vi "CLASS - Generate2DTrain.vi"(8 "error in":errorcluster, 11 "Local":T6={"Parameters"={"Plot"=refnum, "Data"={"Split"={"X Train"=[], "X Test"=[], "Y Train"=[], "Y Test"=[]}, "Predict"=[]}, "Display"={"Choice"=enum."All", "Indexe"={"X"=0, "Y"=0}}, "Property"={"Train Style"=enum."Full circle", "Test OK Style"=enum."Full square", "Label Color"=[8978528, 4367871, 1985280], "Test NO OK"={"Style"=enum."Cross", "Color"=16716800}}}, "2D Array"=[], "Rating 2D Array"=[], "Point ID"=[], "GoodPredict"=0}) -> (0 "error out":errorcluster, 3 "Local Out":T6)   [LabVIEW 2020]
doc: "Generate 2D graph"
uses:
  Controls/2DParameters.ctl
  _Controls/Datas.ctl
  _Controls/PointPropertyMultipleLabel.ctl
  _Controls/Style.ctl
  _Controls/2DData.ctl
types:
  T1 = typedef "2DParameters.ctl" = cluster{"Plot":refnum<vi>, "Data":T2, "Display":cluster{"Choice":enum16{"All", "Train", "Test"}, "Indexe":cluster{"X":i32, "Y":i32}}, "Property":T3}
  T2 = typedef "Datas.ctl" = cluster{"Split":cluster{"X Train":dbl[][], "X Test":dbl[][], "Y Train":dbl[][], "Y Test":dbl[][]}, "Predict":dbl[][]}
  T3 = typedef "PointPropertyMultipleLabel.ctl" = cluster{"Train Style":T4, "Test OK Style":T4, "Label Color":u32[], "Test NO OK":cluster{"Style":T4, "Color":u32}}
  T4 = typedef "Style.ctl" = enum16{"Empty circle", "Full circle", "Empty square", "Full square", "Cross"}
  T5 = typedef "2DData.ctl" = cluster{"Tag":i32, "X":dbl[], "Y":dbl[]}
  T6 = cluster{"Parameters":T1, "2D Array":cluster{"X":dbl[], "Y":dbl[]}[], "Rating 2D Array":T5[], "Point ID":cluster{"DataUse":enum16{"Dataset", "Train", "Test"}, "Color":u32}[], "GoodPredict":i32}
  T7 = cluster{"DataUse":enum16{"Dataset", "Train", "Test"}, "Color":u32}
  T8 = cluster{"X Train":dbl[][], "X Test":dbl[][], "Y Train":dbl[][], "Y Test":dbl[][]}
  T9 = cluster{"DataUse":enum16{"Dataset", "Train", "Test"}, "Color":u32}[]
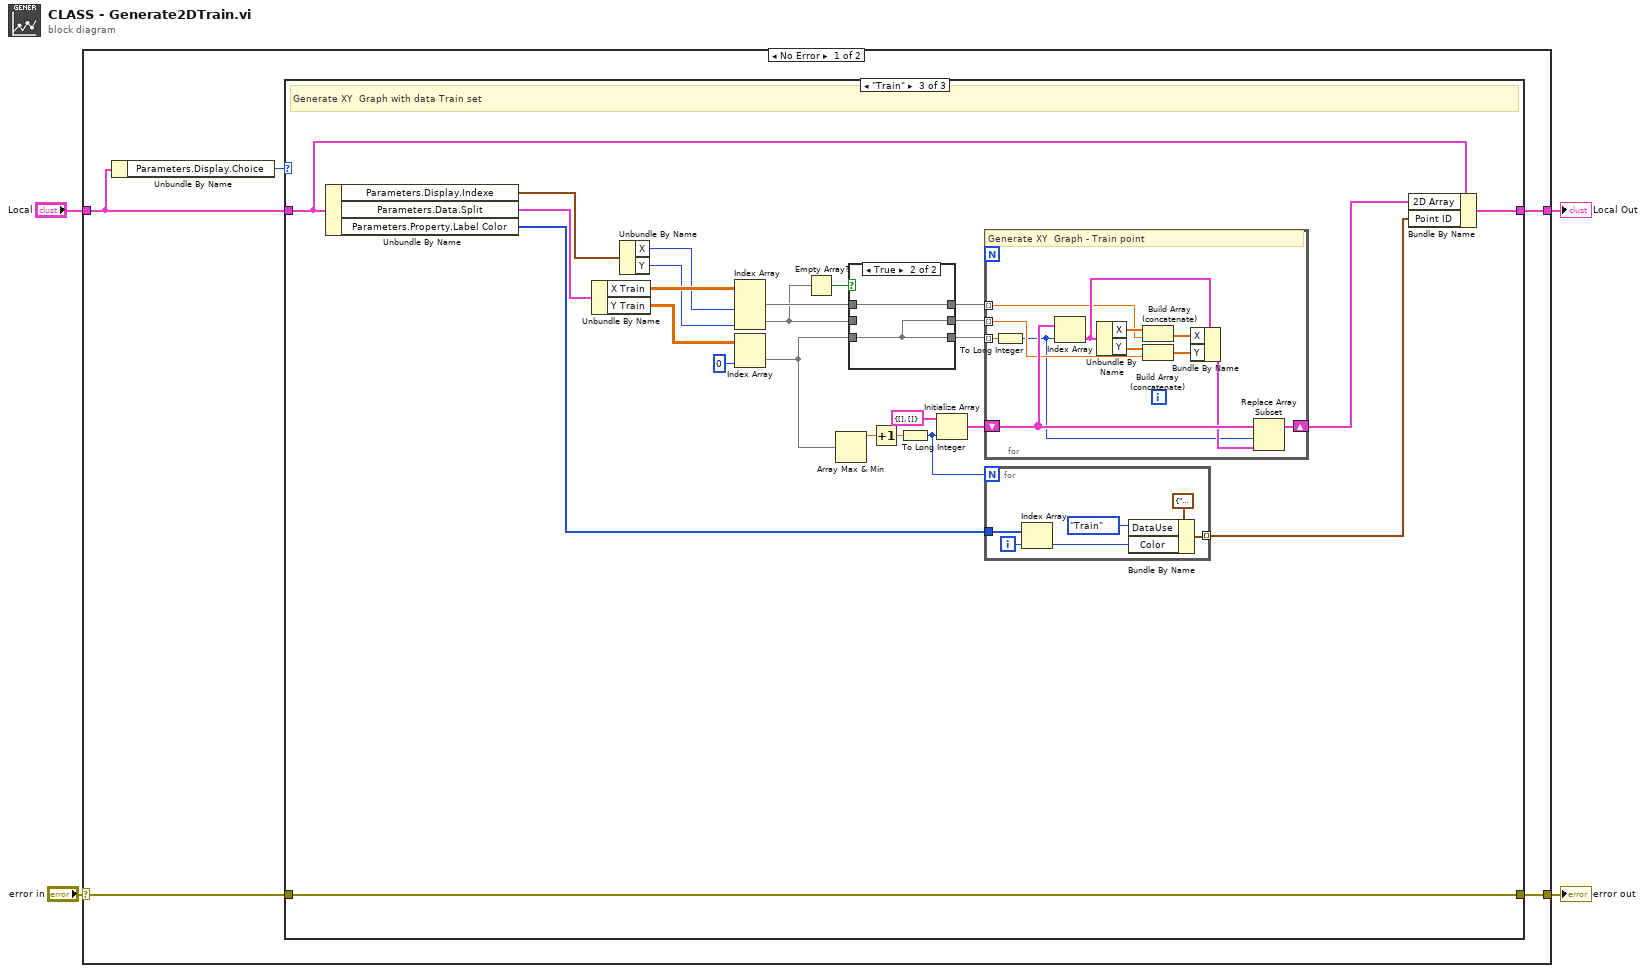
[diagram p0: block diagram]
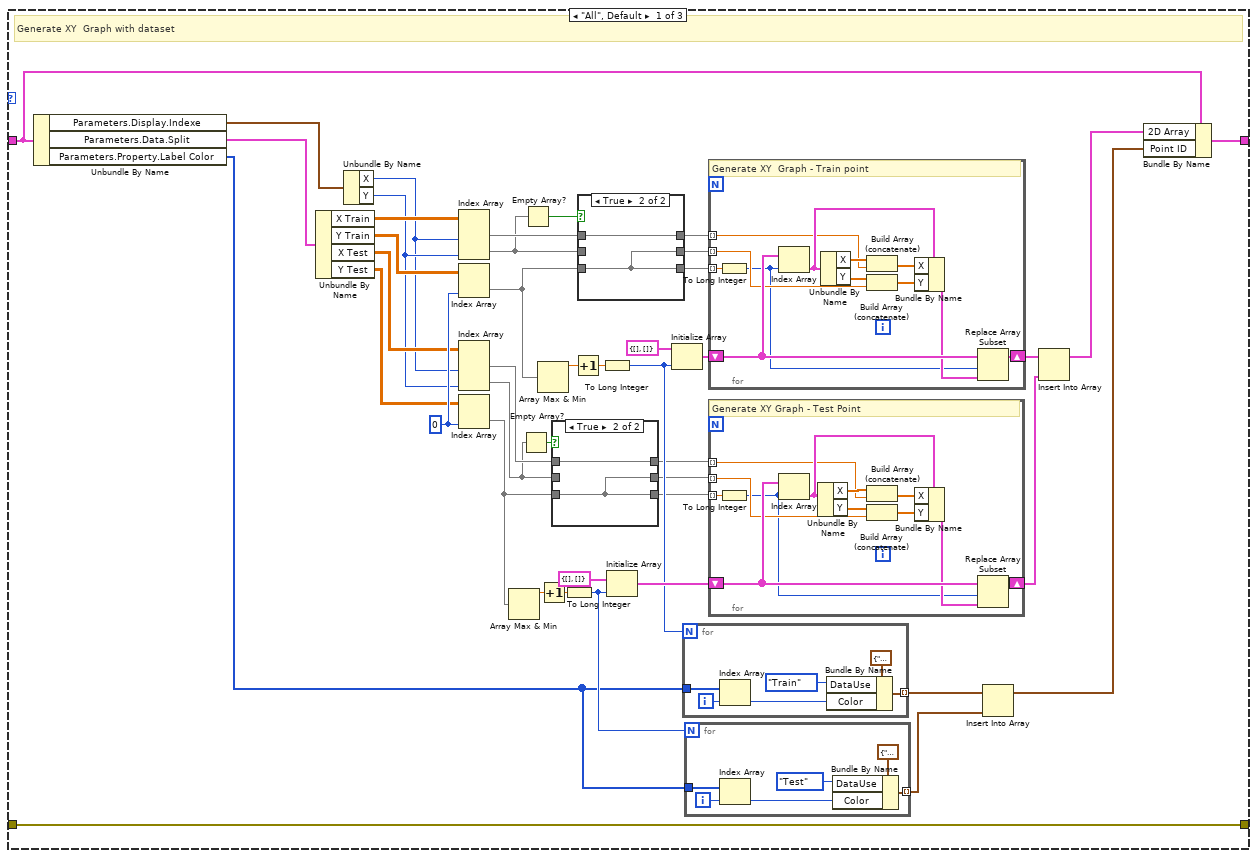
[diagram p2: hidden frame]
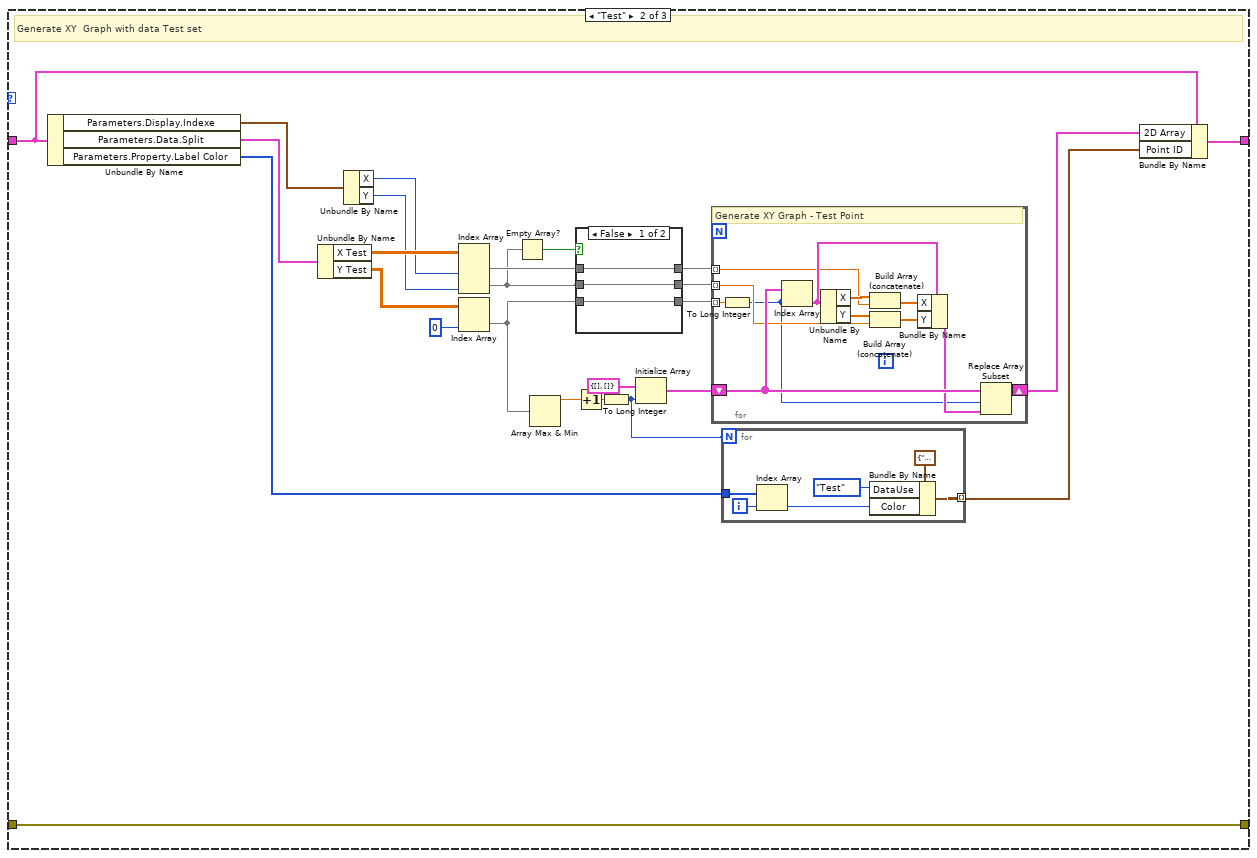
[diagram p5: hidden frame]
diagram:
  n1 = case shown="No Error" "error in" {
    selector: "error in" -> [w7 w195]
    tunnel: "Local" -> [w8 w196]
    tunnel: [w6 w196] -> w1
    tunnel: [w5 w195] -> w3
    frame No Error {
      n2 = Unbundle By Name(w8) -> ("Parameters.Display.Choice"=w9:enum16{"All", "Train", "Test"})
      n3 = case shown="\"Train\"" w9 {
        tunnel: w7 -> [w11 w102 w150]
        tunnel: w8 -> [w34 w113 w162]
        tunnel: [w33 w112 w161] -> w6
        tunnel: [w11 w102 w150] -> w5
        frame "All", Default {
          w41 = 0 ("index of element")
          # "Generate XY  Graph with dataset"
          n4 = Unbundle By Name(w34) -> ("Parameters.Display.Indexe"=w12:cluster{"X":i32, "Y":i32}, "Parameters.Data.Split"=w52:T8, "Parameters.Property.Label Color"=w10:u32[])
          n5 = Unbundle By Name(w52) -> ("X Train"=w40:dbl[][], "Y Train"=w39:dbl[][], "X Test"=w38:dbl[][], "Y Test"=w37:dbl[][])
          n6 = Unbundle By Name(w12) -> ("X"=w35:i32, "Y"=w36:i32)
          n7 = Index Array(array=w40, index (col) #1=w35, index (col) #2=w36) -> (element #1=w26:dbl[], element #2=w21:dbl[])  [unwired: 2 in]
          n8 = Index Array(array=w39, index (col)=w41) -> (element=w23:dbl[])  [unwired: 1 in]
          n9 = Index Array(array=w38, index (col) #1=w35, index (col) #2=w36) -> (element #1=w19:dbl[], element #2=w14:dbl[])  [unwired: 2 in]
          n10 = Index Array(array=w37, index (col)=w41) -> (element=w15:dbl[])  [unwired: 1 in]
          n11 = Array Max & Min(array=w15) -> (max value=w50:dbl)  [unwired: 3 out]
          n12 = Empty Array?(array=w14) -> (empty?=w13:bool)
          n13 = Empty Array?(array=w21) -> (empty?=w20:bool)
          n14 = Array Max & Min(array=w23) -> (max value=w45:dbl)  [unwired: 3 out]
          n15 = Increment(x=w50) -> (x+1=w51:dbl)
          n16 = case shown="True" w13 {
            tunnel: w19 -> [w55 w57]
            tunnel: [w55 w57] -> w18
            tunnel: w14 -> [w54 _]
            tunnel: [w54 w56] -> w17
            tunnel: w15 -> [w53 w56]
            tunnel: [w53 w56] -> w16
            frame False {
            }
            frame True {
            }
          }
          n17 = To Long Integer(number=w51) -> (32bit integer=w30:i32)
          n18 = Increment(x=w45) -> (x+1=w44:dbl)
          n19 = case shown="True" w20 {
            tunnel: w26 -> [w60 w62]
            tunnel: [w60 w62] -> w25
            tunnel: w21 -> [w59 _]
            tunnel: [w59 w61] -> w24
            tunnel: w23 -> [w58 w61]
            tunnel: [w58 w61] -> w22
            frame False {
            }
            frame True {
            }
          }
          n20 = To Long Integer(number=w44) -> (32bit integer=w31:i32)
          n21 = Initialize Array(cluster{"X":dbl[], "Y":dbl[]} {"X"=[], "Y"=[]} ("element"), w30) -> (w48:cluster{"X":dbl[], "Y":dbl[]}[])
          n22 = Initialize Array(cluster{"X":dbl[], "Y":dbl[]} {"X"=[], "Y"=[]} ("element"), w31) -> (w43:cluster{"X":dbl[], "Y":dbl[]}[])
          n23 = for {
            N: w31 -> [_]
            tunnel: [w74] -> w29 mode=indexing
            tunnel: w10 -> [w70]
            i -> [w71]
            n24 = Index Array(array=w70, index=w71) -> (element=w69:u32)
            n25 = Bundle By Name(cluster=T7 {"DataUse"=enum."Train", "Color"=0}, "DataUse"=enum16{"Dataset", "Train", "Test"}."Train", "Color"=w69) -> (w74:T7)
          }
          n26 = for {
            N: w30 -> [_]
            tunnel: [w68] -> w28 mode=indexing
            tunnel: w10 -> [w65]
            i -> [w64]
            n27 = Index Array(array=w65, index=w64) -> (element=w63:u32)
            n28 = Bundle By Name(cluster=T7 {"DataUse"=enum."Train", "Color"=0}, "DataUse"=enum16{"Dataset", "Train", "Test"}."Test", "Color"=w63) -> (w68:T7)
          }
          n29 = for {
            tunnel: w24 -> [w78] mode=indexing
            tunnel: w25 -> [w76] mode=indexing
            tunnel: w22 -> [w80] mode=indexing
            shift-right: [w82] -> w47
            shift-left: w43 -> [w83]
            # "Generate XY  Graph - Train point"
            n30 = To Long Integer(number=w80) -> (32bit integer=w75:i32)
            n31 = Index Array(array=w83, index=w75) -> (element=w86:cluster{"X":dbl[], "Y":dbl[]})
            n32 = Unbundle By Name(w86) -> ("X"=w77:dbl[], "Y"=w79:dbl[])
            n33 = Build Array (concatenate)(w77, w76) -> (w85:dbl[])
            n34 = Build Array (concatenate)(w79, w78) -> (w84:dbl[])
            n35 = Bundle By Name(cluster=w86, "X"=w85, "Y"=w84) -> (w81:cluster{"X":dbl[], "Y":dbl[]})
            n36 = Replace Array Subset(array=w83, new element=w81, index=w75) -> (w82:cluster{"X":dbl[], "Y":dbl[]}[])
          }
          n37 = for {
            tunnel: w17 -> [w90] mode=indexing
            tunnel: w18 -> [w88] mode=indexing
            tunnel: w16 -> [w92] mode=indexing
            shift-right: [w94] -> w46
            shift-left: w48 -> [w95]
            # "Generate XY Graph - Test Point"
            n38 = To Long Integer(number=w92) -> (32bit integer=w87:i32)
            n39 = Index Array(array=w95, index=w87) -> (element=w98:cluster{"X":dbl[], "Y":dbl[]})
            n40 = Unbundle By Name(w98) -> ("X"=w89:dbl[], "Y"=w91:dbl[])
            n41 = Build Array (concatenate)(w89, w88) -> (w97:dbl[])
            n42 = Build Array (concatenate)(w91, w90) -> (w96:dbl[])
            n43 = Bundle By Name(cluster=w98, "X"=w97, "Y"=w96) -> (w93:cluster{"X":dbl[], "Y":dbl[]})
            n44 = Replace Array Subset(array=w95, new element=w93, index=w87) -> (w94:cluster{"X":dbl[], "Y":dbl[]}[])
          }
          n45 = Insert Into Array(array=w29, new element=w28) -> (w27:T9)  [unwired: 1 in]
          n46 = Insert Into Array(array=w47, new element=w46) -> (w32:cluster{"X":dbl[], "Y":dbl[]}[])  [unwired: 1 in]
          n47 = Bundle By Name(cluster=w34, "2D Array"=w32, "Point ID"=w27) -> (w33:T6)
        }
        frame "Test" {
          # "Generate XY  Graph with data Test set"
          n48 = Unbundle By Name(w113) -> ("Parameters.Display.Indexe"=w103:cluster{"X":i32, "Y":i32}, "Parameters.Data.Split"=w123:T8, "Parameters.Property.Label Color"=w99:u32[])
          n49 = Unbundle By Name(w123) -> ("X Test"=w117:dbl[][], "Y Test"=w116:dbl[][])
          n50 = Unbundle By Name(w103) -> ("X"=w114:i32, "Y"=w115:i32)
          n51 = Index Array(array=w117, index (col) #1=w114, index (col) #2=w115) -> (element #1=w109:dbl[], element #2=w105:dbl[])  [unwired: 2 in]
          n52 = Index Array(array=w116, index (col)=0 ("index of element")) -> (element=w104:dbl[])  [unwired: 1 in]
          n53 = Empty Array?(array=w105) -> (empty?=w110:bool)
          n54 = Array Max & Min(array=w104) -> (max value=w121:dbl)  [unwired: 3 out]
          n55 = case shown="False" w110 {
            tunnel: w109 -> [w132 w134]
            tunnel: [w132 w134] -> w108
            tunnel: w105 -> [w131 _]
            tunnel: [w131 w133] -> w107
            tunnel: w104 -> [w130 w133]
            tunnel: [w130 w133] -> w106
            frame False {
            }
            frame True {
            }
          }
          n56 = Increment(x=w121) -> (x+1=w122:dbl)
          n57 = To Long Integer(number=w122) -> (32bit integer=w100:i32)
          n58 = Initialize Array(cluster{"X":dbl[], "Y":dbl[]} {"X"=[], "Y"=[]} ("element"), w100) -> (w119:cluster{"X":dbl[], "Y":dbl[]}[])
          n59 = for {
            tunnel: w107 -> [w138] mode=indexing
            tunnel: w108 -> [w136] mode=indexing
            tunnel: w106 -> [w140] mode=indexing
            shift-right: [w142] -> w111
            shift-left: w119 -> [w143]
            # "Generate XY Graph - Test Point"
            n60 = To Long Integer(number=w140) -> (32bit integer=w135:i32)
            n61 = Index Array(array=w143, index=w135) -> (element=w146:cluster{"X":dbl[], "Y":dbl[]})
            n62 = Unbundle By Name(w146) -> ("X"=w137:dbl[], "Y"=w139:dbl[])
            n63 = Build Array (concatenate)(w137, w136) -> (w145:dbl[])
            n64 = Build Array (concatenate)(w139, w138) -> (w144:dbl[])
            n65 = Bundle By Name(cluster=w146, "X"=w145, "Y"=w144) -> (w141:cluster{"X":dbl[], "Y":dbl[]})
            n66 = Replace Array Subset(array=w143, new element=w141, index=w135) -> (w142:cluster{"X":dbl[], "Y":dbl[]}[])
          }
          n67 = for {
            N: w100 -> [_]
            tunnel: [w129] -> w101 mode=indexing
            tunnel: w99 -> [w126]
            i -> [w125]
            n68 = Index Array(array=w126, index=w125) -> (element=w124:u32)
            n69 = Bundle By Name(cluster=T7 {"DataUse"=enum."Train", "Color"=0}, "DataUse"=enum16{"Dataset", "Train", "Test"}."Test", "Color"=w124) -> (w129:T7)
          }
          n70 = Bundle By Name(cluster=w113, "2D Array"=w111, "Point ID"=w101) -> (w112:T6)
        }
        frame "Train" {
          # "Generate XY  Graph with data Train set"
          n71 = Unbundle By Name(w162) -> ("Parameters.Display.Indexe"=w151:cluster{"X":i32, "Y":i32}, "Parameters.Data.Split"=w171:T8, "Parameters.Property.Label Color"=w147:u32[])
          n72 = Unbundle By Name(w171) -> ("X Train"=w166:dbl[][], "Y Train"=w165:dbl[][])
          n73 = Unbundle By Name(w151) -> ("X"=w163:i32, "Y"=w164:i32)
          n74 = Index Array(array=w166, index (col) #1=w163, index (col) #2=w164) -> (element #1=w155:dbl[], element #2=w152:dbl[])  [unwired: 2 in]
          n75 = Index Array(array=w165, index (col)=0 ("disabled index (col)")) -> (element=w154:dbl[])  [unwired: 1 in]
          n76 = Empty Array?(array=w152) -> (empty?=w153:bool)
          n77 = Array Max & Min(array=w154) -> (max value=w170:dbl)  [unwired: 3 out]
          n78 = case shown="True" w153 {
            tunnel: w155 -> [w180 w182]
            tunnel: [w180 w182] -> w158
            tunnel: w152 -> [w179 _]
            tunnel: [w179 w181] -> w157
            tunnel: w154 -> [w178 w181]
            tunnel: [w178 w181] -> w156
            frame False {
            }
            frame True {
            }
          }
          n79 = Increment(x=w170) -> (x+1=w169:dbl)
          n80 = To Long Integer(number=w169) -> (32bit integer=w148:i32)
          n81 = Initialize Array(cluster{"X":dbl[], "Y":dbl[]} {"X"=[], "Y"=[]} ("element"), w148) -> (w168:cluster{"X":dbl[], "Y":dbl[]}[])
          n82 = for {
            tunnel: w157 -> [w186] mode=indexing
            tunnel: w158 -> [w184] mode=indexing
            tunnel: w156 -> [w188] mode=indexing
            shift-right: [w190] -> w160
            shift-left: w168 -> [w191]
            # "Generate XY  Graph - Train point"
            n83 = To Long Integer(number=w188) -> (32bit integer=w183:i32)
            n84 = Index Array(array=w191, index=w183) -> (element=w194:cluster{"X":dbl[], "Y":dbl[]})
            n85 = Unbundle By Name(w194) -> ("X"=w185:dbl[], "Y"=w187:dbl[])
            n86 = Build Array (concatenate)(w185, w184) -> (w193:dbl[])
            n87 = Build Array (concatenate)(w187, w186) -> (w192:dbl[])
            n88 = Bundle By Name(cluster=w194, "X"=w193, "Y"=w192) -> (w189:cluster{"X":dbl[], "Y":dbl[]})
            n89 = Replace Array Subset(array=w191, new element=w189, index=w183) -> (w190:cluster{"X":dbl[], "Y":dbl[]}[])
          }
          n90 = for {
            N: w148 -> [_]
            tunnel: [w177] -> w149 mode=indexing
            tunnel: w147 -> [w173]
            i -> [w174]
            n91 = Index Array(array=w173, index=w174) -> (element=w172:u32)
            n92 = Bundle By Name(cluster=T7 {"DataUse"=enum."Train", "Color"=0}, "DataUse"=enum16{"Dataset", "Train", "Test"}."Train", "Color"=w172) -> (w177:T7)
          }
          n93 = Bundle By Name(cluster=w162, "2D Array"=w160, "Point ID"=w149) -> (w161:T6)
        }
      }
    }
    frame Error {
    }
  }
  "error out" <- w3
  "Local Out" <- w1
